vi "pulsenoisevar.vi"(0 "input current derivative":sgl[](array[numeric]) format="%.2f", 1 "input time":sgl[](array[numeric]) format="%.2f", 2 "start time":sgl=0.0001 format="%.2e", 3 "end time":dbl=0.02 format="%.2f") -> (5 "standard deviation of 2nd derivative":ext=838.4002871488872 format="%.10f")   [LabVIEW 2016]
uses:
  <vilib>/Analysis/2dsp.llb/Derivative x(t).vi
  <vilib>/Analysis/NI_AALBase.lvlib
  <vilib>/Analysis/NI_AALPro.lvlib
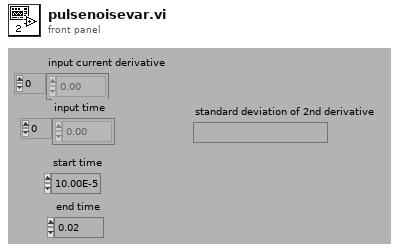
[diagram p1: front panel]
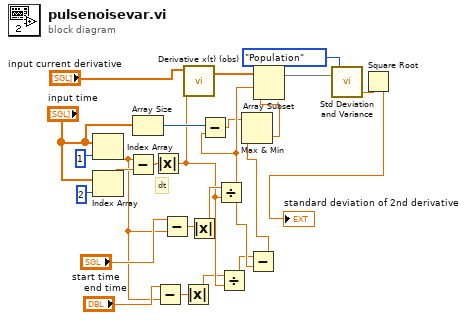
[diagram p0: block diagram]
diagram:
  # "dt"
  n1 = Index Array(array="input time", index=1) -> (element=w7:sgl)
  n2 = Index Array(array="input time", index=2) -> (element=w23:sgl)
  n3 = Subtract(x=w7, y=w23) -> (x-y=w22:sgl)
  n4 = Array Size(array="input time") -> (size(s)=w16:i32)
  n5 = Absolute Value(x=w22) -> (abs(x)=w5:sgl)
  n6 = Subtract(x="end time", y=w7) -> (x-y=w6:dbl)
  n7 = Subtract(x="start time", y=w7) -> (x-y=w20:sgl)
  n8 = Absolute Value(x=w6) -> (abs(x)=w4:dbl)
  n9 = call <vilib>:"Derivative x(t) (obs).vi"("dt"=w5, "X"="input current derivative") -> ("dX/dt"=w14:dbl[])  [unwired: 2 in, 1 out]
  n10 = Absolute Value(x=w20) -> (abs(x)=w19:sgl)
  n11 = Divide(x=w19, y=w5) -> (x/y=w15:sgl)
  n12 = Subtract(x=w16, y=w15) -> (x-y=w10:sgl)
  n13 = Divide(x=w4, y=w5) -> (x/y=w3:dbl)
  n14 = Subtract(x=w3, y=w15) -> (x-y=w2:dbl)
  n15 = Max & Min(x=w10, y=w2) -> (min(x,y)=w9:dbl)  [unwired: 1 out]
  n16 = Array Subset(array=w14, index=w15, length=w9) -> (w13:dbl[])
  n17 = call <vilib>:"Std Deviation and Variance.vi"("X"=w13, "Weighting (Sample)"=enum16{"Sample", "Population"}."Population") -> ("variance"=w12:dbl)  [unwired: 2 out]
  n18 = Square Root(x=w12) -> (sqrt(x)=→"standard deviation of 2nd derivative":dbl)
